vi "Create Message Channels Section.vi"(8 "error in (no error)":errorcluster, 11 "Message in":T1 format="%.0x") -> (0 "error out":errorcluster, 1 "Message Channels Section out":T1 format="%.0x", 3 "Message out":T1 format="%.0x")   [LabVIEW 2018, in "Instrument Addon Scripting API.lvlib"]
uses:
  Instrument Addon Scripting API.lvlib
  <vilib>/NI Veristand/Custom Device API/Custom Device Item Ref.ctl
  Addon/Addon Shared/SubVIs/Constants.vi
  Addon/Addon Shared/Instrument Addon Shared.lvlib
  <vilib>/NI Veristand/Custom Device API/Custom Device API.lvlib
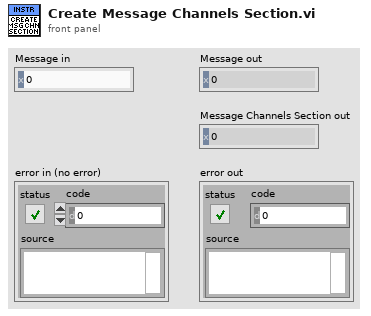
[diagram p1: front panel]
types:
  T1 = typedef "Custom Device API.lvlib/Custom Device Item Ref.ctl" = u64
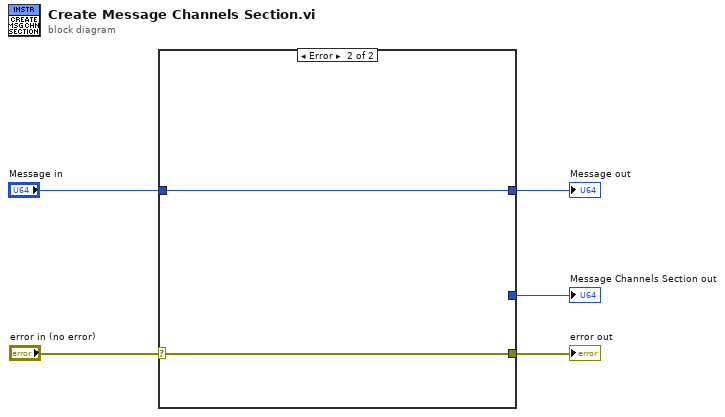
[diagram p0: block diagram]
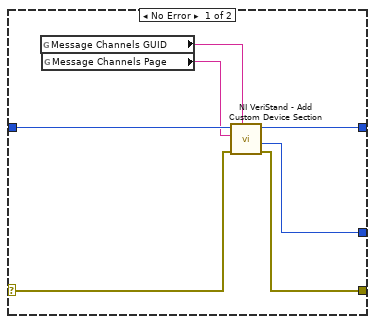
[diagram p2: hidden frame]
diagram:
  n1 = case shown="Error" "error in (no error)" {
    selector: "error in (no error)" -> [w6 w14]
    tunnel: [w12 w13] -> w5
    tunnel: "Message in" -> [w11 w13]
    tunnel: [w10 _] -> w3
    tunnel: [w9 w14] -> w2
    frame No Error {
      n2 = global read "Constants.vi" "Message Channels GUID"() -> (w8:string)
      n3 = global read "Constants.vi" "Message Channels Page"() -> (w7:string)
      n4 = call <vilib>:"NI VeriStand - Add Custom Device Section.vi"("GUID (Default Section)"=w8, "error in (no error)"=w6, "Section Name"=w7, "Parent Ref in"=w11) -> ("error out"=w9:errorcluster, "Section Ptr"=w10:T1, "Parent Ref out"=w12:T1)  [unwired: 4 in, 1 out]
    }
    frame Error {
    }
  }
  "Message out" <- w5
  "Message Channels Section out" <- w3
  "error out" <- w2
